vi "lvEtherbone.socket_close.vi"(0 "eb_socket_ID":i32, 5 "error in (no error)":errorcluster) -> (13 "eb_status":T1 items=["EB_SUCCESS"=1, "EB_OK"=0, "EB_FAIL"=-1, "EB_ADDRESS"=-2, "EB_WIDTH"=-3, "EB_OVERFLOW"=-4, "EB_ENDIAN"=-5, "EB_BUSY"=-6, "EB_TIMEOUT"=-7, "EB_OOM"=-8, "EB_ABI"=-9, "EB_SEGFAULT"=-10], 19 "error out":errorcluster)   [LabVIEW 2012, in "lvEtherbone.lvlib"]
doc: "/* Close the Etherbone socket.\n * Any use of the socket after successful close will probably segfault!\n *\n * Return codes:\n * OK - successfully closed the socket and freed memory\n * BUSY - there are open devices on this socket\n */\nEB_PUBLIC\neb_status_t eb_socket_close(eb_socket_t socket);"
uses:
  lvEtherbone.lvlib
  lvEtherbone.lveb_status_t.ctl
  libetherbone.so
panel:
  in  "eb_status_t":T1 items=["EB_SUCCESS"=1, "EB_OK"=0, "EB_FAIL"=-1, "EB_ADDRESS"=-2, "EB_WIDTH"=-3, "EB_OVERFLOW"=-4, "EB_ENDIAN"=-5, "EB_BUSY"=-6, "EB_TIMEOUT"=-7, "EB_OOM"=-8, "EB_ABI"=-9, "EB_SEGFAULT"=-10]
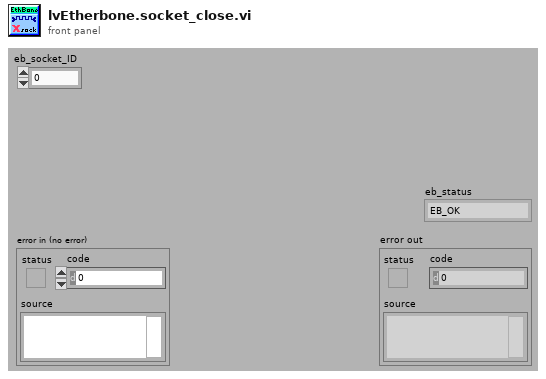
[diagram p1: front panel]
types:
  T1 = typedef "lvEtherbone.lvlib/lvEtherbone.lveb_status_t.ctl" = i32
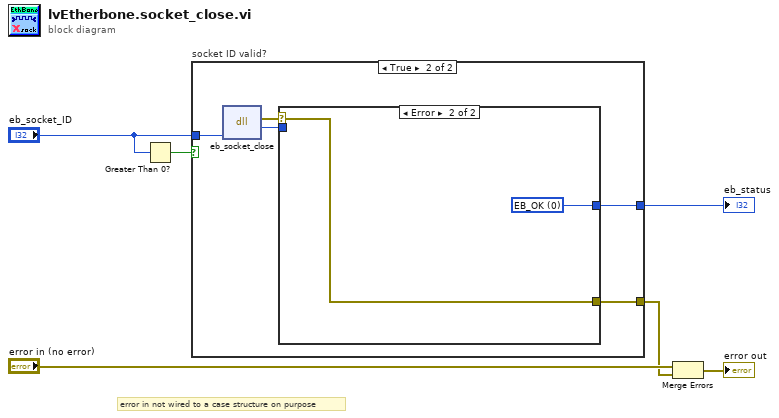
[diagram p0: block diagram]
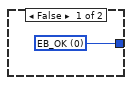
[diagram p2: hidden frame]
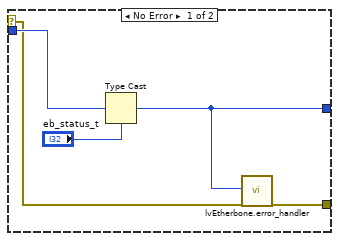
[diagram p3: hidden frame]
diagram:
  # "error in not wired to a case structure on purpose"
  n1 = Greater Than 0?(x="eb_socket_ID") -> (x > 0?=w1:bool)
  n2 = case "socket ID valid?" shown="True" w1 {
    tunnel: [w7 w12] -> w6
    tunnel: "eb_socket_ID" -> [_ w11]
    tunnel: [_ w8] -> w3
    frame False {
      w7 = T1 0 items=["EB_SUCCESS"=1, "EB_OK"=0, "EB_FAIL"=-1, "EB_ADDRESS"=-2, "EB_WIDTH"=-3, "EB_OVERFLOW"=-4, "EB_ENDIAN"=-5, "EB_BUSY"=-6, "EB_TIMEOUT"=-7, "EB_OOM"=-8, "EB_ABI"=-9, "EB_SEGFAULT"=-10] ("eb_status_t")
    }
    frame True {
      n3 = dll-call lib="libetherbone.so" fn="eb_socket_close"("eb_socket_ID"=w11) -> (error out=w9:errorcluster, "eb_status"=w10:i32)  [unwired: 4 in, 1 out]
      n4 = case shown="Error" w9 {
        selector: w9 -> [w13 w19]
        tunnel: w10 -> [w17 _]
        tunnel: [w15 w18] -> w12
        tunnel: [w14 w19] -> w8
        frame No Error {
          n5 = Type Cast(type="eb_status_t", x=w17) -> (*(type *) &x=w15:T1)
          n6 = call "lvEtherbone.error_handler.vi"("eb_status"=w15, "error in"=w13) -> ("error out"=w14:errorcluster)  [unwired: 17 in]
        }
        frame Error {
          w18 = T1 0 items=["EB_SUCCESS"=1, "EB_OK"=0, "EB_FAIL"=-1, "EB_ADDRESS"=-2, "EB_WIDTH"=-3, "EB_OVERFLOW"=-4, "EB_ENDIAN"=-5, "EB_BUSY"=-6, "EB_TIMEOUT"=-7, "EB_OOM"=-8, "EB_ABI"=-9, "EB_SEGFAULT"=-10] ("eb_status_t")
        }
      }
    }
  }
  "eb_status" <- w6
  n7 = Merge Errors("error in (no error)", w3) -> (→"error out":errorcluster)
